vi "Configure SMU Voltage Limit Tracking.vi"(8 "error in (no error)":errorcluster {"code" format="%.0x"}, 9 "Enable Voltage Limit Tracking (False)":bool, 10 "Channel Name (1)":string="1", 11 "VISA resource name":refnum<visa-resource-name>) -> (0 "error out":errorcluster {"code" format="%.0x"}, 3 "VISA resource name out":refnum<visa-resource-name>)   [LabVIEW 2018, in "Agilent N6700 Series.lvlib"]
doc: "Sets the voltage limit tracking state. \n\n<b>Notes:</b>\n(1) This VI only applies to model N6784A.\n(2) The output protection priority must be set to current in <b>Configure Output Regulation.vi</b>."
uses:
  Agilent N6700 Series.lvlib
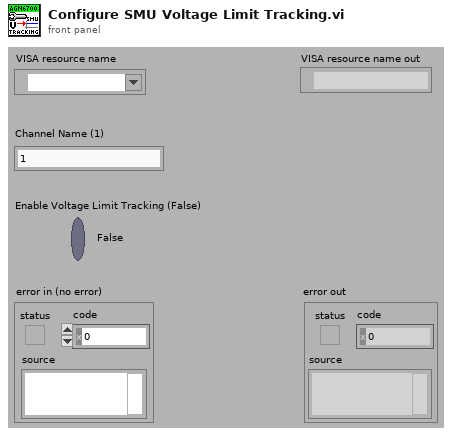
[diagram p1: front panel]
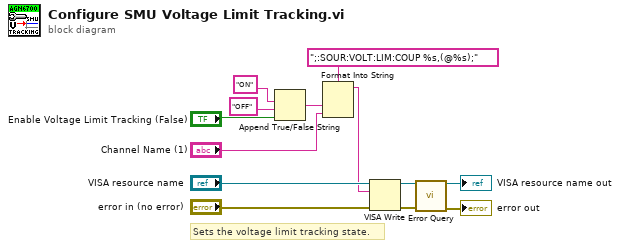
[diagram p0: block diagram]
diagram:
  # "Sets the voltage limit tracking state."
  n1 = Append True/False String(1:"Enable Voltage Limit Tracking (False)", 2:"OFF", 3:"ON") -> (0:w5:string)  [unwired: 1 in]
  n2 = Format Into String(format string=";:SOUR:VOLT:LIM:COUP %s,(@%s);", w5, "Channel Name (1)") -> (resulting string=w2:string)  [unwired: 2 in, 1 out]
  n3 = VISA Write(VISA resource name="VISA resource name", write buffer=w2, error in (no error)="error in (no error)") -> (VISA resource name out=w9:refnum<visa-resource-name>, error out=w8:errorcluster)  [unwired: 1 out]
  n4 = call "Error Query.vi"("VISA resource name"=w9, "error in (no error)"=w8) -> ("VISA resource name out"=→"VISA resource name out":refnum<visa-resource-name>, "error out"=→"error out":errorcluster)  [unwired: 10 in, 2 out]
